vi "Write System Status Ref.vi"(8 "error in (no error)":errorcluster, 10 "System Status Ref":refnum<vi>, 11 "System Actor in":refnum<class "System Actor.lvclass">) -> (0 "error out":errorcluster, 3 "System Actor out":refnum<class "System Actor.lvclass">)   [LabVIEW 2014, in "Robot Actors.lvlib" / "System Actor.lvlib" / "System Actor.lvclass"]
uses:
  System Actor.lvclass
  System Status.ctl
  Command/Command Class/Command Status.ctl
  Command/Command Class/Command States.ctl
  Command Processor/Command Processor Class/Command Processor Status.ctl
  Command Processor/Command Processor Class/Command Processor States.ctl
  System Actor.lvclass/System Actor.ctl
  Command/Command Class/Command.lvclass
  Command Processor/Command Processor Class/Command Processor.lvclass
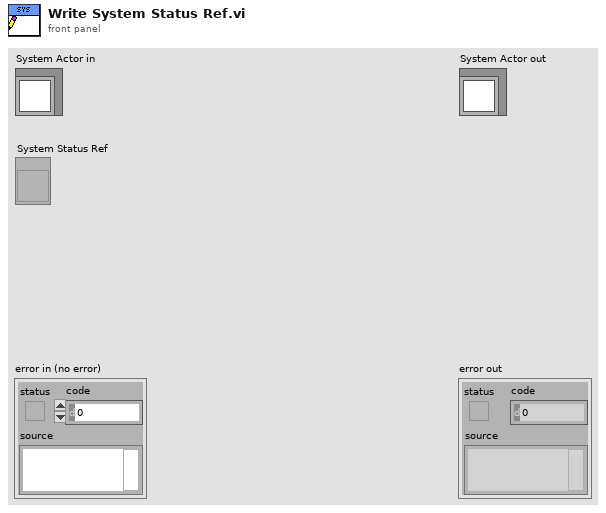
[diagram p1: front panel]
types:
  T1 = typedef "Robot Actors.lvlib/System Actor.lvlib/System Actor.lvclass/System Status.ctl" = cluster{"Instance Name":string, "Command Status":T2, "System Start Time":timestamp, "Next Command ID":dbl, "Command Processor Status":T4}
  T2 = typedef "Robot Actors.lvlib/Command.lvlib/Command.lvclass/Command Status.ctl" = cluster{"Command Name":string, "Command Start Time":timestamp, "Command End Time":timestamp, "Is Command Finished?":bool, "Command ID":dbl, "Command State":T3}
  T3 = typedef "Robot Actors.lvlib/Command.lvlib/Command.lvclass/Command States.ctl" = enum16{"Unknown", "Started", "Stopped", "Finished"}
  T4 = typedef "Robot Actors.lvlib/Command Processor.lvlib/Command Processor.lvclass/Command Processor Status.ctl" = cluster{"Next Command ID":dbl, "Current Command Status":T2, "Previous Command Status ":T2, "Command Processor State":T5, "Last Status Update":timestamp}
  T5 = typedef "Robot Actors.lvlib/Command Processor.lvlib/Command Processor.lvclass/Command Processor States.ctl" = enum16{"Unknown", "No Command", "Running Command"}
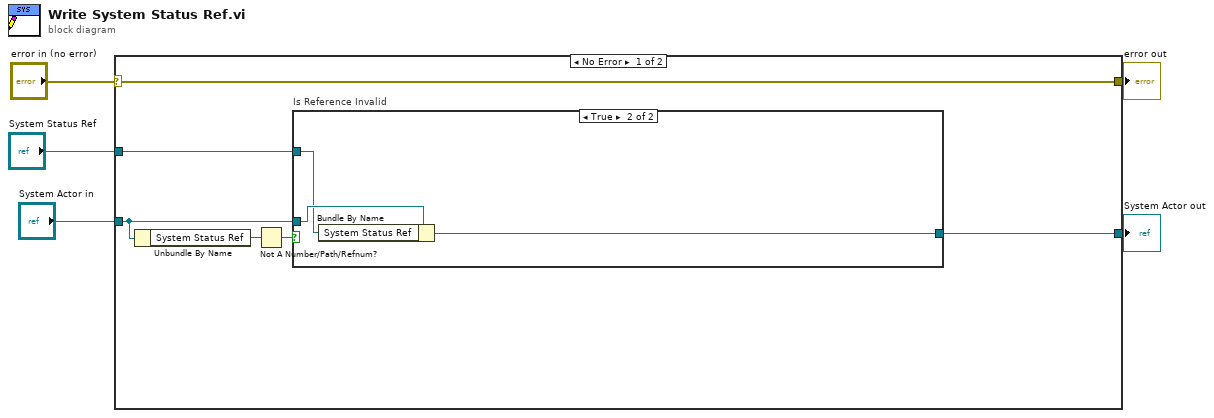
[diagram p0: block diagram]
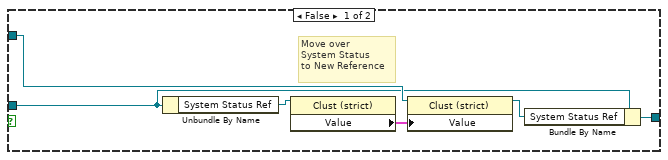
[diagram p2: hidden frame]
diagram:
  n1 = case shown="No Error" "error in (no error)" {
    selector: "error in (no error)" -> [w11 w21]
    tunnel: [w11 w21] -> w4
    tunnel: [w10 w22] -> w2
    tunnel: "System Actor in" -> [w8 w22]
    tunnel: "System Status Ref" -> [w9 _]
    frame No Error {
      n2 = Unbundle By Name(w8) -> ("System Status Ref"=w7:refnum<vi>)
      n3 = Not A Number/Path/Refnum?(number/path/refnum=w7) -> (NaN/Path/Refnum?=w6:bool)
      n4 = case "Is Reference Invalid" shown="True" w6 {
        tunnel: w8 -> [w14 w20]
        tunnel: [w13 w19] -> w10
        tunnel: w9 -> [w16 w18]
        frame False {
          # "Move over\nSystem Status\nto New Reference"
          n5 = Unbundle By Name(w14) -> ("System Status Ref"=w17:refnum<vi>)
          n6 = property class="Clust (strict)"(reference=w17) -> ("Value"=w15:T1)  [unwired: 1 in, 2 out]
          n7 = property class="Clust (strict)"(reference=w16, "Value"=w15) -> (reference out=w12:refnum<vi>)  [unwired: 1 in, 1 out]
          n8 = Bundle By Name(cluster=w14, "System Status Ref"=w12) -> (w13:refnum<class "System Actor.lvclass">)
        }
        frame True {
          n9 = Bundle By Name(cluster=w20, "System Status Ref"=w18) -> (w19:refnum<class "System Actor.lvclass">)
        }
      }
    }
    frame Error {
    }
  }
  "error out" <- w4
  "System Actor out" <- w2
